vi "Q Metadata (SubVI).vi"(11 "Measurement Data":T1) -> ()   [LabVIEW 2015]
uses:
  Controls (FPGA)/SPLINE Measurement Data.ctl
  <vilib>/rvi/interface/RandomDataEmulation/niFpgaRandomDataHandleErrors.vi
  <vilib>/rvi/DataTransferAndStorage/Container/XNode/niFpgaContainer.xnode
  <vilib>/rvi/interface/RandomDataEmulation/nirviRandomDataFpgaReadWriteTemplate.vi
  <vilib>/rvi/FIFO/Fifo_Resource/nirvififoEmulationWrite.vi
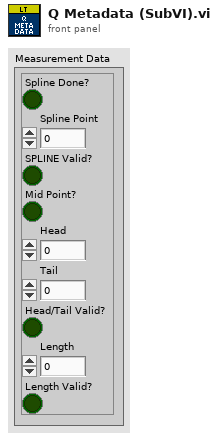
[diagram p1: front panel]
types:
  T1 = typedef "SPLINE Measurement Data.ctl" = cluster{"Spline Done?":bool, "Spline Point":u32, "SPLINE Valid?":bool, "Mid Point?":bool, "Head":u32, "Tail":u32, "Head/Tail Valid?":bool, "Length":u16, "Length Valid?":bool}
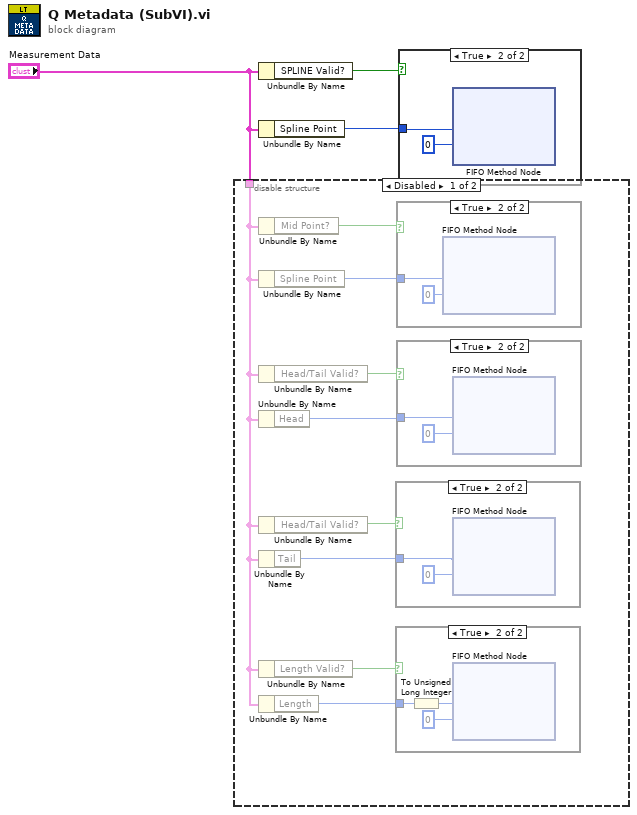
[diagram p0: block diagram]
diagram:
  n1 = disable-structure shown="Disabled" {
    disable-tunnel: "Measurement Data" -> [w12 _]
    frame Disabled {
      n2 = Unbundle By Name(w12) -> ("Mid Point?"=w4:bool)
      n3 = Unbundle By Name(w12) -> ("Spline Point"=w5:u32)
      n4 = Unbundle By Name(w12) -> ("Head/Tail Valid?"=w6:bool)
      n5 = Unbundle By Name(w12) -> ("Head"=w7:u32)
      n6 = Unbundle By Name(w12) -> ("Head/Tail Valid?"=w8:bool)
      n7 = Unbundle By Name(w12) -> ("Tail"=w9:u32)
      n8 = Unbundle By Name(w12) -> ("Length Valid?"=w11:bool)
      n9 = Unbundle By Name(w12) -> ("Length"=w10:u16)
      n10 = case shown="True" w8 {
        tunnel: w9 -> [_ w16]
        frame False {
        }
        frame True {
          n11 = xnode ("FIFO Method Node")("Element"=w16, "Timeout"=0) -> ()  [unwired: 1 in, 2 out]
        }
      }
      n12 = case shown="True" w11 {
        tunnel: w10 -> [_ w14]
        frame False {
        }
        frame True {
          n13 = To Unsigned Long Integer(number=w14) -> (unsigned 32bit integer=w13:u32)
          n14 = xnode ("FIFO Method Node")("Element"=w13, "Timeout"=0) -> ()  [unwired: 1 in, 2 out]
        }
      }
      n15 = case shown="True" w4 {
        tunnel: w5 -> [_ w20]
        frame False {
        }
        frame True {
          n16 = xnode ("FIFO Method Node")("Element"=w20, "Timeout"=0) -> ()  [unwired: 1 in, 2 out]
        }
      }
      n17 = case shown="True" w6 {
        tunnel: w7 -> [_ w18]
        frame False {
        }
        frame True {
          n18 = xnode ("FIFO Method Node")("Element"=w18, "Timeout"=0) -> ()  [unwired: 1 in, 2 out]
        }
      }
    }
    frame Enabled {
    }
  }
  n19 = Unbundle By Name("Measurement Data") -> ("SPLINE Valid?"=w1:bool)
  n20 = Unbundle By Name("Measurement Data") -> ("Spline Point"=w2:u32)
  n21 = case shown="True" w1 {
    tunnel: w2 -> [_ w22]
    frame False {
    }
    frame True {
      n22 = xnode ("FIFO Method Node")("Element"=w22, "Timeout"=0) -> ()  [unwired: 1 in, 2 out]
    }
  }
